vi "Auton File Loader.vi"   [LabVIEW 2015]
uses:
  Common Code/Auton File Lists.ctl
  Robot Global Data.vi
types:
  T1 = typedef "Auton File Lists.ctl" = cluster{"Current Queue":string, "General Scripts":string, "Defense Scripts":string, "Movement Scripts":string}
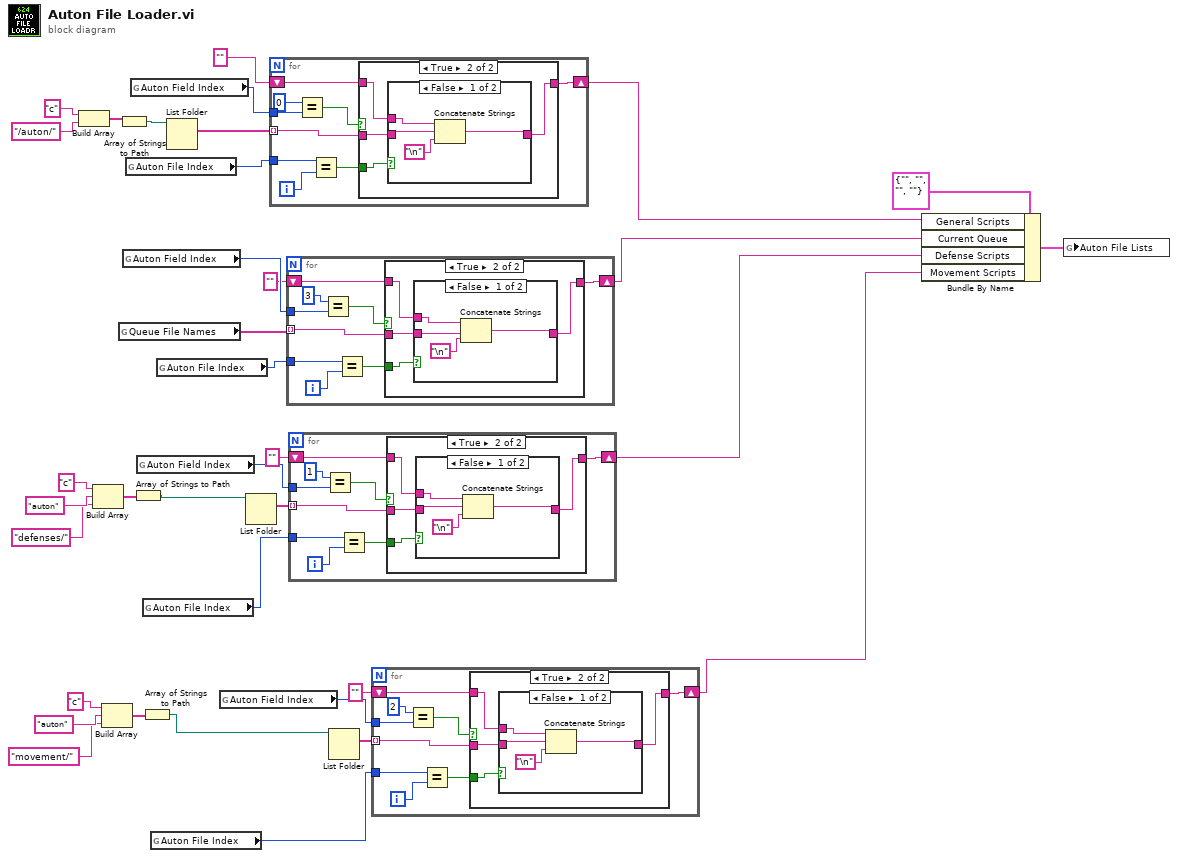
[diagram p0: block diagram]
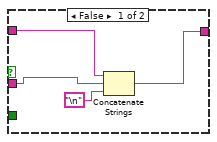
[diagram p2: hidden frame]
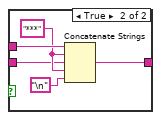
[diagram p3: hidden frame]
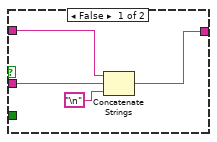
[diagram p4: hidden frame]
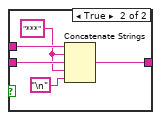
[diagram p5: hidden frame]
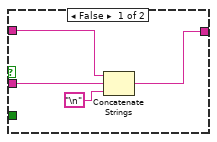
[diagram p6: hidden frame]
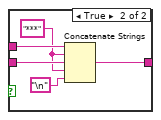
[diagram p7: hidden frame]
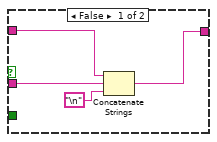
[diagram p8: hidden frame]
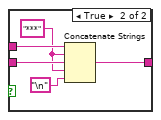
[diagram p9: hidden frame]
diagram:
  n1 = Build Array("c", "/auton/") -> (w12:string[])
  n2 = Build Array("c", "auton", "defenses/" ("element")) -> (w8:string[])
  n3 = Build Array("c", "auton", "movement/" ("element")) -> (w4:string[])
  n4 = Array of Strings to Path(0:w12) -> (2:w11:path)  [unwired: 1 in]
  n5 = global read "Robot Global Data.vi" "Queue File Names"() -> (w24:string[])
  n6 = global read "Robot Global Data.vi" "Auton Field Index"() -> (w26:i32)
  n7 = global read "Robot Global Data.vi" "Auton File Index"() -> (w34:i32)
  n8 = global read "Robot Global Data.vi" "Auton Field Index"() -> (w35:i32)
  n9 = Array of Strings to Path(0:w8) -> (2:w6:path)  [unwired: 1 in]
  n10 = global read "Robot Global Data.vi" "Auton Field Index"() -> (w31:i32)
  n11 = Array of Strings to Path(0:w4) -> (2:w2:path)  [unwired: 1 in]
  n12 = global read "Robot Global Data.vi" "Auton File Index"() -> (w23:i32)
  n13 = global read "Robot Global Data.vi" "Auton File Index"() -> (w22:i32)
  n14 = global read "Robot Global Data.vi" "Auton File Index"() -> (w25:i32)
  n15 = List Folder(path=w11) -> (filenames=w36:string[])  [unwired: 3 in, 3 out]
  n16 = global read "Robot Global Data.vi" "Auton Field Index"() -> (w30:i32)
  n17 = List Folder(path=w6) -> (filenames=w32:string[])  [unwired: 3 in, 3 out]
  n18 = for {
    tunnel: w36 -> [w38] mode=indexing
    tunnel: w35 -> [w45]
    tunnel: w34 -> [w42]
    shift-right: [w37] -> w19
    shift-left: "" -> [w39]
    i -> [w41]
    n19 = Equal?(x=0, y=w45) -> (x = y?=w43:bool)
    n20 = Equal?(x=w42, y=w41) -> (x = y?=w40:bool)
    n21 = case shown="True" w43 {
      tunnel: w40 -> [_ w53]
      tunnel: w39 -> [w49 w52]
      tunnel: w38 -> [w48 w51]
      tunnel: [w46 w50] -> w37
      frame False {
        n22 = Concatenate Strings(w49, w48, "\n") -> (w46:string)
      }
      frame True {
        n23 = case shown="False" w53 {
          tunnel: w52 -> [w57 w62]
          tunnel: w51 -> [w56 w61]
          tunnel: [w54 w58] -> w50
          frame False {
            n24 = Concatenate Strings(w57, w56, "\n") -> (w54:string)
          }
          frame True {
            w60 = "***"
            n25 = Concatenate Strings(w62, w60, w61, w60, "\n") -> (w58:string)
          }
        }
      }
    }
  }
  n26 = for {
    tunnel: w24 -> [w66] mode=indexing
    shift-right: [w65] -> w27
    shift-left: "" -> [w67]
    tunnel: w26 -> [w64]
    tunnel: w25 -> [w63]
    i -> [w69]
    n27 = Equal?(x=3, y=w64) -> (x = y?=w70:bool)
    n28 = Equal?(x=w63, y=w69) -> (x = y?=w68:bool)
    n29 = case shown="True" w70 {
      tunnel: w68 -> [_ w79]
      tunnel: w67 -> [w75 w78]
      tunnel: w66 -> [w72 w77]
      tunnel: [w73 w76] -> w65
      frame False {
        n30 = Concatenate Strings(w75, w72, "\n") -> (w73:string)
      }
      frame True {
        n31 = case shown="False" w79 {
          tunnel: w78 -> [w83 w88]
          tunnel: w77 -> [w80 w84]
          tunnel: [w81 w85] -> w76
          frame False {
            n32 = Concatenate Strings(w83, w80, "\n") -> (w81:string)
          }
          frame True {
            w87 = "***"
            n33 = Concatenate Strings(w88, w87, w84, w87, "\n") -> (w85:string)
          }
        }
      }
    }
  }
  n34 = for {
    tunnel: w32 -> [w92] mode=indexing
    shift-right: [w91] -> w28
    shift-left: "" -> [w93]
    tunnel: w31 -> [w90]
    tunnel: w23 -> [w89]
    i -> [w95]
    n35 = Equal?(x=1, y=w90) -> (x = y?=w96:bool)
    n36 = Equal?(x=w89, y=w95) -> (x = y?=w94:bool)
    n37 = case shown="True" w96 {
      tunnel: w94 -> [_ w105]
      tunnel: w93 -> [w101 w104]
      tunnel: w92 -> [w100 w103]
      tunnel: [w98 w102] -> w91
      frame False {
        n38 = Concatenate Strings(w101, w100, "\n") -> (w98:string)
      }
      frame True {
        n39 = case shown="False" w105 {
          tunnel: w104 -> [w109 w114]
          tunnel: w103 -> [w108 w113]
          tunnel: [w106 w110] -> w102
          frame False {
            n40 = Concatenate Strings(w109, w108, "\n") -> (w106:string)
          }
          frame True {
            w112 = "***"
            n41 = Concatenate Strings(w114, w112, w113, w112, "\n") -> (w110:string)
          }
        }
      }
    }
  }
  n42 = List Folder(path=w2) -> (filenames=w29:string[])  [unwired: 3 in, 3 out]
  n43 = for {
    tunnel: w29 -> [w118] mode=indexing
    shift-right: [w117] -> w20
    shift-left: "" -> [w119]
    tunnel: w30 -> [w116]
    tunnel: w22 -> [w115]
    i -> [w121]
    n44 = Equal?(x=2, y=w116) -> (x = y?=w122:bool)
    n45 = Equal?(x=w115, y=w121) -> (x = y?=w120:bool)
    n46 = case shown="True" w122 {
      tunnel: w120 -> [_ w131]
      tunnel: w119 -> [w127 w130]
      tunnel: w118 -> [w126 w129]
      tunnel: [w124 w128] -> w117
      frame False {
        n47 = Concatenate Strings(w127, w126, "\n") -> (w124:string)
      }
      frame True {
        n48 = case shown="False" w131 {
          tunnel: w130 -> [w135 w140]
          tunnel: w129 -> [w134 w139]
          tunnel: [w132 w136] -> w128
          frame False {
            n49 = Concatenate Strings(w135, w134, "\n") -> (w132:string)
          }
          frame True {
            w138 = "***"
            n50 = Concatenate Strings(w140, w138, w139, w138, "\n") -> (w136:string)
          }
        }
      }
    }
  }
  n51 = Bundle By Name(cluster=T1 {"Current Queue"="", "General Scripts"="", "Defense Scripts"="", "Movement Scripts"=""} ("Auton File Lists"), "General Scripts"=w19, "Current Queue"=w27, "Defense Scripts"=w28, "Movement Scripts"=w20) -> (w21:T1)
  n52 = global write "Robot Global Data.vi" "Auton File Lists"(w21) -> ()
